vi "NormalizeProfile.vi"(11 "Z profile":dbl[](array[numeric])) -> (3 "Array":dbl[](array[numeric]))   [LabVIEW 2011]
uses:
  <vilib>/Analysis/5stat.llb/RMS (DBL).vi
  <vilib>/Analysis/NI_AALBase.lvlib
  <vilib>/Analysis/NI_AALPro.lvlib
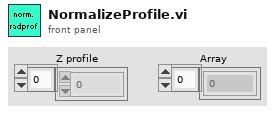
[diagram p1: front panel]
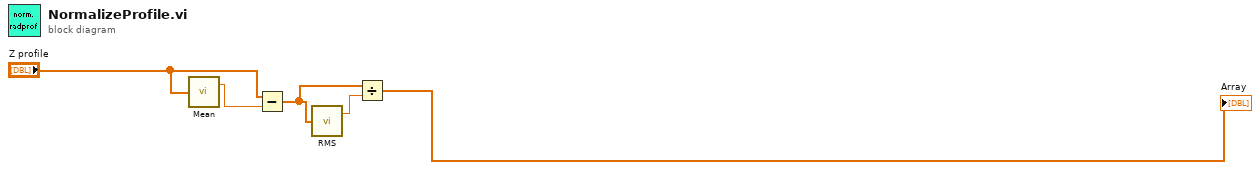
[diagram p0: block diagram]
diagram:
  n1 = call <vilib>:"Mean.vi"("X"="Z profile") -> ("mean"=w2:dbl)  [unwired: 1 out]
  n2 = Subtract(x="Z profile", y=w2) -> (x-y=w3:dbl[])
  n3 = call-poly <vilib>:"RMS.vi"("X"=w3) -> ("rms value"=w4:dbl)  [unwired: 1 out]
  n4 = Divide(x=w3, y=w4) -> (x/y=→"Array":dbl[])
